vi "ziMDSStart.vi"(0 "Master":string="dev", 5 "Slaves":string[](array[string])=["dev"]) -> (4 "Handle Out":T1 {"Handle" format="0x%08x"; "Conn" format="0x%08x"}, 6 "ModHandle Out":T2 {"ModHandle" format="0x%08x"; "Conn" format="0x%08x"}, 8 "MDS_Devices":string[](array[string]), 10 "Status":dbl, 14 "Message":string, 15 "Error Out":errorcluster)   [LabVIEW 2018, in "Zurich Instruments LabOne.lvlib"]
doc: "Enabels multiDeviceSync (MDS) on the Master and Slave devices and returns the status of the MDS.\nNote: You have stop the MDS once done (multiDeviceSyncModule/start,0), run ziModClear.vi and run ziClose.vi to clean up all connections."
uses:
  Zurich Instruments LabOne.lvlib
  Modules/ziModSetValueDoubleArray.vi
  Modules/ziModSetValueBinary.vi
  Modules/ziModSetValueDouble.vi
  Modules/ziModGetNodeValueDouble.vi
  Modules/ziModGetNodeValueString.vi
  Modules/ziTypeModEnum.ctl
  Configure/ziSetValueBinary.vi
  Modules/ziTypeModHandle.ctl
  ziTypeHandle.ctl
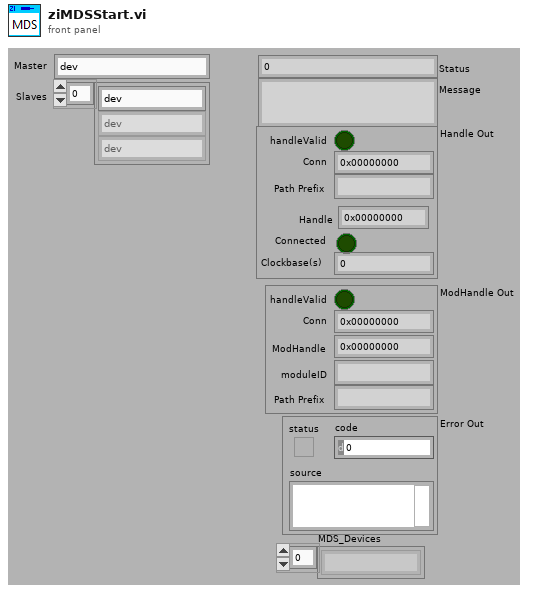
[diagram p1: front panel]
types:
  T1 = typedef "Zurich Instruments LabOne.lvlib/ziTypeHandle.ctl" = cluster{"handleValid":bool, "Conn":u64, "Path Prefix":string, "Handle":u64, "Connected":bool, "Clockbase(s)":dbl}
  T2 = typedef "Zurich Instruments LabOne.lvlib/ziTypeModHandle.ctl" = cluster{"handleValid":bool, "Conn":u64, "ModHandle":u64, "moduleID":string, "Path Prefix":string}
  T3 = typedef "Zurich Instruments LabOne.lvlib/ziTypeModEnum.ctl" = u16
  T4 = typedef "Zurich Instruments LabOne.lvlib/ziTypeDisovery.ctl" = cluster{"timestamp":u64, "deviceid":string, "devicetype":string, "serveraddress":string, "serverport":u32, "apilevel":u32, "discoverable":bool, "interface":string, "connected":string, "available":bool, "owner":string, "status":string, "options ":string, "serverversion":string}
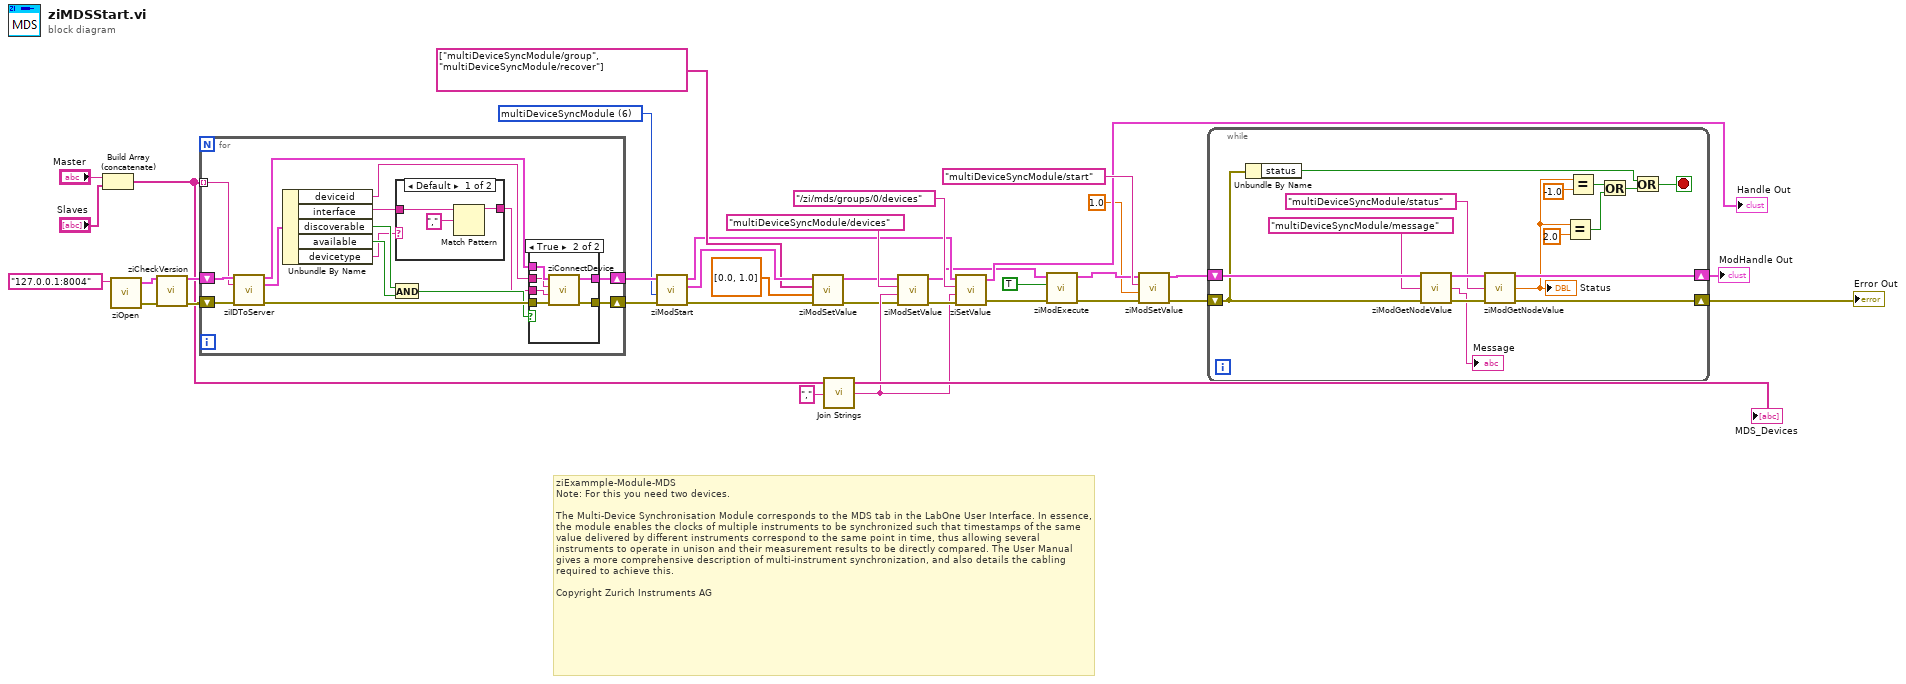
[diagram p0: block diagram]
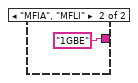
[diagram p2: hidden frame]
diagram:
  w24 = T3 6 items=["sweep", "scopeModule", "dataAcquisitionModule", "pidAdvisor", "awgModule", "impedanceModule", "multiDeviceSyncModule", "zoomFFT", "trigger", "deviceSettings", "record"] ("module Id")
  # "ziExammple-Module-MDS\nNote: For this you need two devices.\n \nThe Multi-Device Synchronisation Module corresponds to the MDS tab in the LabOne User Interface. In essence, the module enables the clocks of multiple instruments to be synchronized such that timestamps of the same value delivered by different instruments correspond to the same point in time, thus allowing several instruments to operate in unison and their measurement results to be directly compared. The User Manual gives a more comprehensive description of multi-instrument synchronization, and also details the cabling required to achieve this.\n\nCopyright Zurich Instruments AG"
  n1 = Build Array (concatenate)("Master", "Slaves") -> (w18:string[])
  "MDS_Devices" <- w18
  n2 = call "ziOpen.vi"("Address"="127.0.0.1:8004") -> ("Error Out"=w21:errorcluster, "HandleOut"=w22:T1)  [unwired: 3 in, 1 out]
  n3 = call "ziCheckVersion.vi"("Handle In"=w22, "Error In"=w21) -> ("Handle Out"=w27:T1, "Error Out"=w26:errorcluster)  [unwired: 11 in, 1 out]
  n4 = for {
    shift-right: [w50] -> w35
    shift-left: w27 -> [w48]
    shift-right: [w49] -> w34
    shift-left: w26 -> [w47]
    tunnel: w18 -> [w43] mode=indexing
    n5 = call "ziIDToServer.vi"("ziHandle In"=w48, "Device ID"=w43, "Error In"=w47) -> ("ziHandle Out"=w46:T1, "ziDiscovery"=w44:T4, "Error Out"=w45:errorcluster)  [unwired: 10 in]
    n6 = Unbundle By Name(w44) -> ("deviceid"=w39:string, "interface"=w37:string, "discoverable"=w42:bool, "available"=w41:bool, "devicetype"=w38:string)
    n7 = And(x=w42, y=w41) -> (x .and. y?=w40:bool)
    n8 = case shown="Default" w38 {
      tunnel: w37 -> [w53 _]
      tunnel: [w51 "1GBE" ("interface")] -> w36
      frame Default {
        n9 = Match Pattern(string=w53, regular expression=",") -> (before substring=w51:string)  [unwired: 1 in, 3 out]
      }
      frame "MFIA", "MFLI" {
      }
    }
    n10 = case shown="True" w40 {
      tunnel: [w56 w62] -> w50
      tunnel: [w55 w61] -> w49
      tunnel: w46 -> [w56 w60]
      tunnel: w45 -> [w55 w59]
      tunnel: w39 -> [_ w58]
      tunnel: w36 -> [_ w57]
      frame False {
      }
      frame True {
        n11 = call "ziConnectDevice.vi"("Error In"=w59, "Device Interface"=w57, "Device Serial"=w58, "Handle In"=w60) -> ("Error Out"=w61:errorcluster, "Handle Out"=w62:T1)  [unwired: 6 in]
      }
    }
  }
  n12 = call "ziModStart.vi"("Error In"=w34, "module Id"=w24, "Handle In"=w35) -> ("Error Out"=w13:errorcluster, "ModHandle Out"=w31:T2, "Handle Out"=w14:T1)  [unwired: 6 in]
  n13 = call-poly "ziModSetValue.vi"("Error In"=w13, "Values"=dbl[] [0.0, 1.0], "Paths"=string[] ["multiDeviceSyncModule/group", "multiDeviceSyncModule/recover"], "ModHandle In"=w31) -> ("Error Out"=w9:errorcluster, "ModHandle Out"=w10:T2)  [unwired: 6 in]
  n14 = call <vilib>:"Join Strings.vi"("Separator (,)"="," ("string"), "Strings In"=w18) -> ("String"=w11:string)  [unwired: 1 in]
  n15 = call-poly "ziModSetValue.vi"("Error In"=w9, "Data"=w11, "Path"="multiDeviceSyncModule/devices", "ModHandle In"=w10) -> ("Error Out"=w12:errorcluster, "ModHandle Out"=w3:T2)  [unwired: 6 in]
  n16 = call-poly "ziSetValue.vi"("Error In"=w12, "Data"=w11, "Path"="/zi/mds/groups/0/devices", "Handle In"=w14) -> ("Error Out"=w8:errorcluster, "Handle Out"=→"Handle Out":T1)  [unwired: 1 in]
  n17 = call "ziModExecute.vi"("Error In"=w8, "Modal (F)"=TRUE, "ziModHandle In"=w3) -> ("Error Out"=w4:errorcluster, "ziModHandle Out"=w6:T2)  [unwired: 5 in, 1 out]
  n18 = call-poly "ziModSetValue.vi"("Error In"=w4, "Value"=1.0, "Path"="multiDeviceSyncModule/start", "ModHandle In"=w6) -> ("Error Out"=w29:errorcluster, "ModHandle Out"=w30:T2)  [unwired: 6 in]
  n19 = while {
    shift-right: [w71] -> w28
    shift-left: w30 -> [w78]
    shift-right: [w72] -> w1
    shift-left: w29 -> [w65]
    stop <- w63 stop-if-true
    n20 = Unbundle By Name(w65) -> ("status"=w66:bool)
    n21 = call-poly "ziModGetNodeValue.vi"("ModHandle In"=w78, "Path"="multiDeviceSyncModule/message", "error in"=w65) -> ("ModHandle Out"=w77:T2, "Value"=→"Message":string, "error out"=w76:errorcluster)  [unwired: 10 in]
    n22 = call-poly "ziModGetNodeValue.vi"("ModHandle In"=w77, "Path"="multiDeviceSyncModule/status", "error in"=w76) -> ("ModHandle Out"=w71:T2, "Value"=w68:dbl, "error out"=w72:errorcluster)  [unwired: 10 in]
    "Status" <- w68
    n23 = Equal?(x=w68, y=2.0) -> (x = y?=w69:bool)
    n24 = Equal?(x=w68, y=-1.0) -> (x = y?=w70:bool)
    n25 = Or(x=w70, y=w69) -> (x .or. y?=w64:bool)
    n26 = Or(x=w66, y=w64) -> (x .or. y?=w63:bool)
  }
  "Error Out" <- w1
  "ModHandle Out" <- w28
